vi "Read Measurements.vi"(11 "Test Framework in":refnum<class "Test Framework.lvclass">) -> (2 "Measurements":refnum<class "Measurement.lvclass">[](array[class]), 3 "Test Framework out":refnum<class "Test Framework.lvclass">)   [LabVIEW 2020, in "Test Framework.lvclass"]
uses:
  Test Framework.lvclass
  Measurements/Measurement.lvclass
  Test Framework.lvclass/Test Framework.ctl
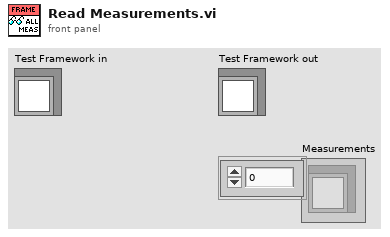
[diagram p1: front panel]
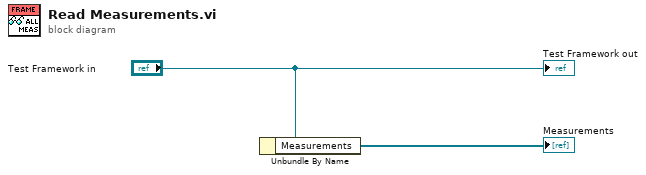
[diagram p0: block diagram]
diagram:
  n1 = Unbundle By Name("Test Framework in") -> ("Measurements"=→"Measurements":refnum<class "Measurement.lvclass">[])
  "Test Framework out" <- "Test Framework in"
